vi "wd_replaceInIndexFindPre.vi"(9 "value index":u64, 10 "RecordInfo":T1[](array[typedef]), 11 "node start index":i32) -> (2 "value index out":u64, 3 "pre node index":i32)   [LabVIEW 2020, in "NI_ExcelFile.lvlib"]
uses:
  <vilib>/express/express shared/NI_ExcelFile/NI_ExcelFile.lvlib
  <vilib>/express/express shared/NI_ExcelFile/Ctrls/wd_recordInfo.ctl
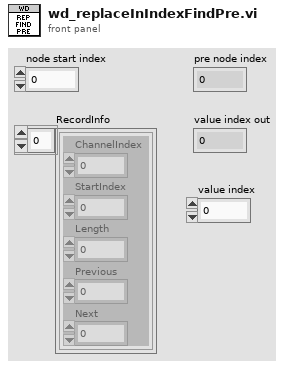
[diagram p1: front panel]
types:
  T1 = typedef "NI_ExcelFile.lvlib/wd_recordInfo.ctl" = cluster{"ChannelIndex":u32, "StartIndex":u64, "Length":u64, "Previous":i32, "Next":i32}
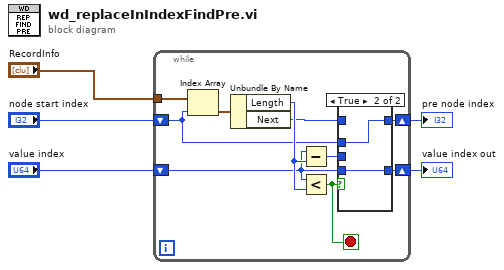
[diagram p0: block diagram]
diagram:
  n1 = while {
    shift-right: [w10] -> w3
    shift-left: "node start index" -> [w9]
    shift-right: [w7] -> w4
    shift-left: "value index" -> [w6]
    tunnel: "RecordInfo" -> [w15]
    stop <- w12 stop-if-true
    n2 = Index Array(array=w15, index=w9) -> (element=w14:T1)
    n3 = Unbundle By Name(w14) -> ("Length"=w13:u64, "Next"=w11:i32)
    n4 = Subtract(x=w6, y=w13) -> (x-y=w8:u64)
    n5 = Less?(x=w6, y=w13) -> (x < y?=w12:bool)
    n6 = case shown="True" w12 {
      tunnel: w11 -> [w17 _]
      tunnel: [w17 w19] -> w10
      tunnel: w9 -> [_ w19]
      tunnel: w8 -> [w16 _]
      tunnel: [w16 w18] -> w7
      tunnel: w6 -> [_ w18]
      frame False {
      }
      frame True {
      }
    }
  }
  "value index out" <- w4
  "pre node index" <- w3
